vi "Data-log-trigger-data.vi"(5 "Trigg?":bool, 7 "Plant to trigg":enum16{"Plant 1", "Plant 2"}(ring), 10 "Scheduler State":T2, 11 "Data cluster in":cluster{"Plant 2":T1, "Plant 1":T1}) -> (3 "Data cluster out":cluster{"Plant 2":T1, "Plant 1":T1})   [LabVIEW 2016]
uses:
  Plant-data.ctl
  Sched_state.ctl
  Plant_info.ctl
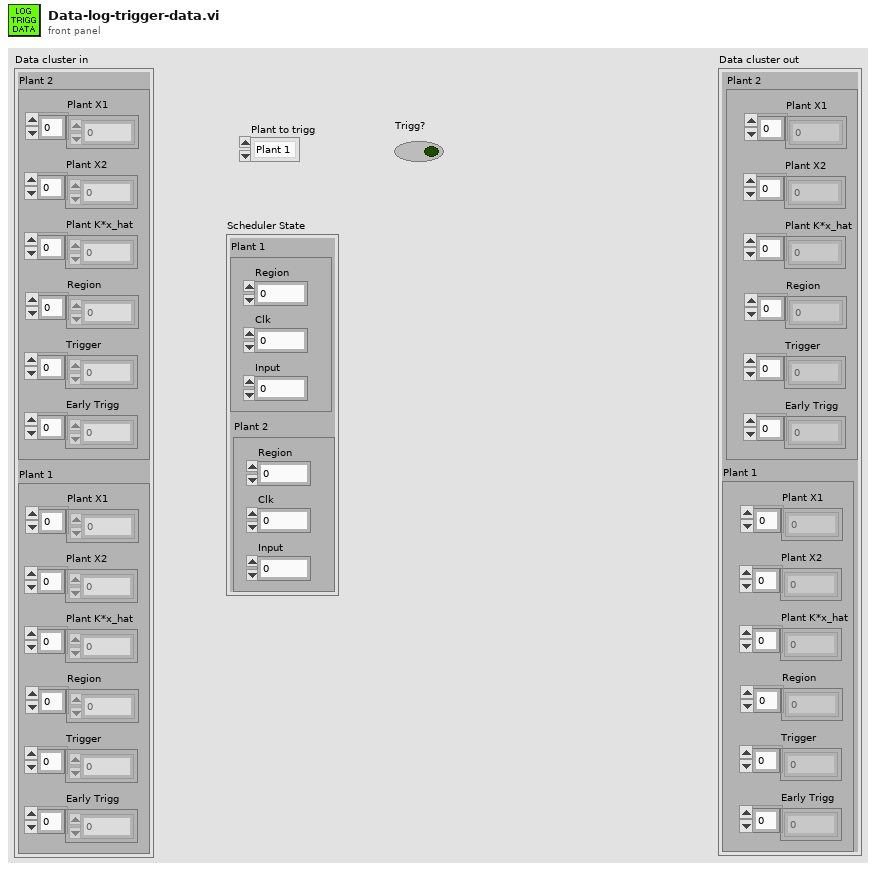
[diagram p1: front panel]
types:
  T1 = typedef "Plant-data.ctl" = cluster{"Plant X1 ":dbl[], "Plant X2":dbl[], "Plant K*x_hat":dbl[], "Region":i32[], "Trigger":i32[], "Early Trigg":i32[]}
  T2 = typedef "Sched_state.ctl" = cluster{"Plant 1":T3, "Plant 2":T3}
  T3 = typedef "Plant_info.ctl" = cluster{"Clk":dbl, "Region":dbl, "Input":dbl}
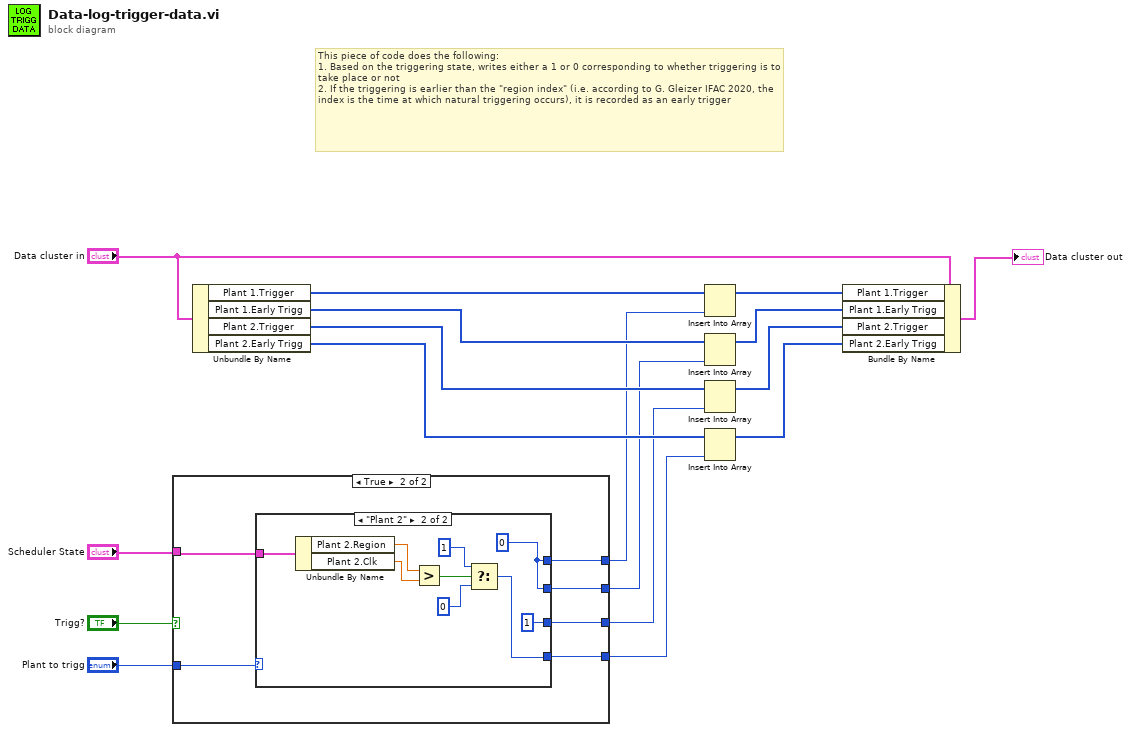
[diagram p0: block diagram]
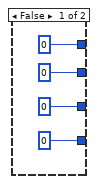
[diagram p2: hidden frame]
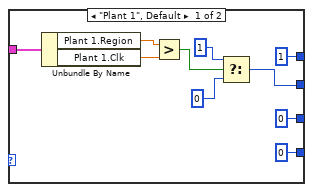
[diagram p3: hidden frame]
diagram:
  # "This piece of code does the following:\n1. Based on the triggering state, writes either a 1 or 0 corresponding to whether triggering is to take place or not\n2. If the triggering is earlier than the \"region index\" (i.e. according to G. Gleizer IFAC 2020, the index is the time at which natural triggering occurs), it is recorded as an early trigger"
  n1 = case shown="True" "Trigg?" {
    tunnel: [0 w25] -> w9
    tunnel: [0 w24] -> w8
    tunnel: [0 w23] -> w7
    tunnel: [0 w22] -> w6
    tunnel: "Plant to trigg" -> [_ w27]
    tunnel: "Scheduler State" -> [_ w26]
    frame False {
    }
    frame True {
      n2 = case shown="\"Plant 2\"" w27 {
        tunnel: w26 -> [w37 w46]
        tunnel: [1 ("f") w38] -> w25
        tunnel: [w29 w38] -> w24
        tunnel: [0 1] -> w23
        tunnel: [0 ("f") w39] -> w22
        frame "Plant 1", Default {
          n3 = Unbundle By Name(w37) -> ("Plant 1.Region"=w30:dbl, "Plant 1.Clk"=w36:dbl)
          n4 = Greater?(x=w30, y=w36) -> (0:w35:bool)
          n5 = Select(t=1, s=w35, f=0) -> (s? t:f=w29:i32)
        }
        frame "Plant 2" {
          w38 = 0 ("f")
          n6 = Unbundle By Name(w46) -> ("Plant 2.Region"=w44:dbl, "Plant 2.Clk"=w43:dbl)
          n7 = Greater?(x=w44, y=w43) -> (0:w42:bool)
          n8 = Select(t=1, s=w42, f=0) -> (s? t:f=w39:i32)
        }
      }
    }
  }
  n9 = Unbundle By Name("Data cluster in") -> ("Plant 1.Trigger"=w16:i32[], "Plant 1.Early Trigg"=w13:i32[], "Plant 2.Trigger"=w12:i32[], "Plant 2.Early Trigg"=w11:i32[])
  n10 = Insert Into Array(array=w16, new element=w9) -> (w15:i32[])  [unwired: 1 in]
  n11 = Insert Into Array(array=w13, new element=w8) -> (w5:i32[])  [unwired: 1 in]
  n12 = Insert Into Array(array=w12, new element=w7) -> (w4:i32[])  [unwired: 1 in]
  n13 = Insert Into Array(array=w11, new element=w6) -> (w3:i32[])  [unwired: 1 in]
  n14 = Bundle By Name(cluster="Data cluster in", "Plant 1.Trigger"=w15, "Plant 1.Early Trigg"=w5, "Plant 2.Trigger"=w4, "Plant 2.Early Trigg"=w3) -> (→"Data cluster out":cluster{"Plant 2":T1, "Plant 1":T1})
